vi "ATSh_InputBandwidth.vi"(9 "Bandwidth":u32, 10 "Channel":u32, 11 "Handle":u32) -> (0 "Return":u32, 3 "Handle_out":u32)   [LabVIEW 2014]
doc: "_____AlazarTech, Scope_____\n\nConfigure the bandwidth.\nHandle input.\n\n\nChannel:\n - A : 0x01\n - B : 0x02\n\nBandwidth:\n - Full : 0x00\n - Reduce : 0x01"
uses:
  ATSApi.dll
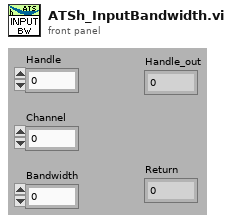
[diagram p1: front panel]
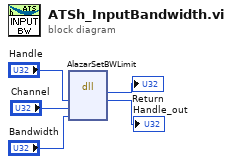
[diagram p0: block diagram]
diagram:
  n1 = dll-call lib="D:/IntensityOCT/trunk/ATSApi.dll" fn="AlazarSetBWLimit"("h"="Handle", "Channel"="Channel", "Bandwidth"="Bandwidth") -> (→"Return":u32, "h"=→"Handle_out":u32)  [unwired: 5 in, 2 out]
